vi "Z900_navX_Internal_UpdateDevice.vi"(8 "error in (no error)":errorcluster, 10 "Interface TypeDefs":T1 {"I2CDevRef"."Device Address" format="%.0x"}, 11 "navX Device":T8={"Interface"={"Protocol"=enum."SERIAL", "Update Rate (4Hz-60Hz)"=4, "navX Open TypeDef"=variant}, "Notify Packet"=refnum, "Loop VI Refnum"=refnum} {"Interface"."Update Rate (4Hz-60Hz)" min=4 max=60 step=1}) -> (0 "error out":errorcluster, 2 "Interface TypeDefs":T1 {"I2CDevRef"."Device Address" format="%.0x"}, 3 "navX Device":T8={"Interface"={"Protocol"=enum."SERIAL", "Update Rate (4Hz-60Hz)"=4, "navX Open TypeDef"=variant}, "Notify Packet"=refnum, "Loop VI Refnum"=refnum} {"Interface"."Update Rate (4Hz-60Hz)" min=4 max=60 step=1})   [LabVIEW 2014, in "navX Library v2.lvlib"]
uses:
  navX Library v2.lvlib
  TypeDefs/Z900_navX_DeviceTypeDef.ctl
  TypeDefs/Z900_navX_ProtocolTypeDef.ctl
  TypeDefs/Z900_navX_NotifyPacketTypeDef.ctl
  TypeDefs/Z900_navX_ActionTypeDef.ctl
  TypeDefs/Z900_navX_InterfaceTypeDef.ctl
  <vilib>/Rock Robotics/WPI/SerialPort/WPI_SerialPortRef.ctl
  <vilib>/Rock Robotics/WPI/I2C/WPI_I2CDevRef.ctl
  <vilib>/Rock Robotics/SystemInterfaces/Typedef/FPGA_TypedefDigitalModule.ctl
  <vilib>/Rock Robotics/SystemInterfaces/i2clib/i2c_bus.ctl
  <vilib>/Rock Robotics/WPI/SPI/WPI_SPIDevRef.ctl
  <vilib>/Rock Robotics/SystemInterfaces/spilib/spi_bus.ctl
  TypeDefs/navX Open TypeDefs/Z900_navX_OpenTypeDef_Serial.ctl
  NI WPI/WPI_SerialPort_USB.ctl
  TypeDefs/Z900_navX_SerialStreamTypeDef.ctl
  TypeDefs/navX Open TypeDefs/Z900_navX_OpenTypeDef_I2C.ctl
  TypeDefs/Z900_navX_DeviceRegisters.ctl
  TypeDefs/navX Open TypeDefs/Z900_navX_OpenTypeDef_SPI.ctl
  NI WPI/NI WPI Serial USB.lvlib
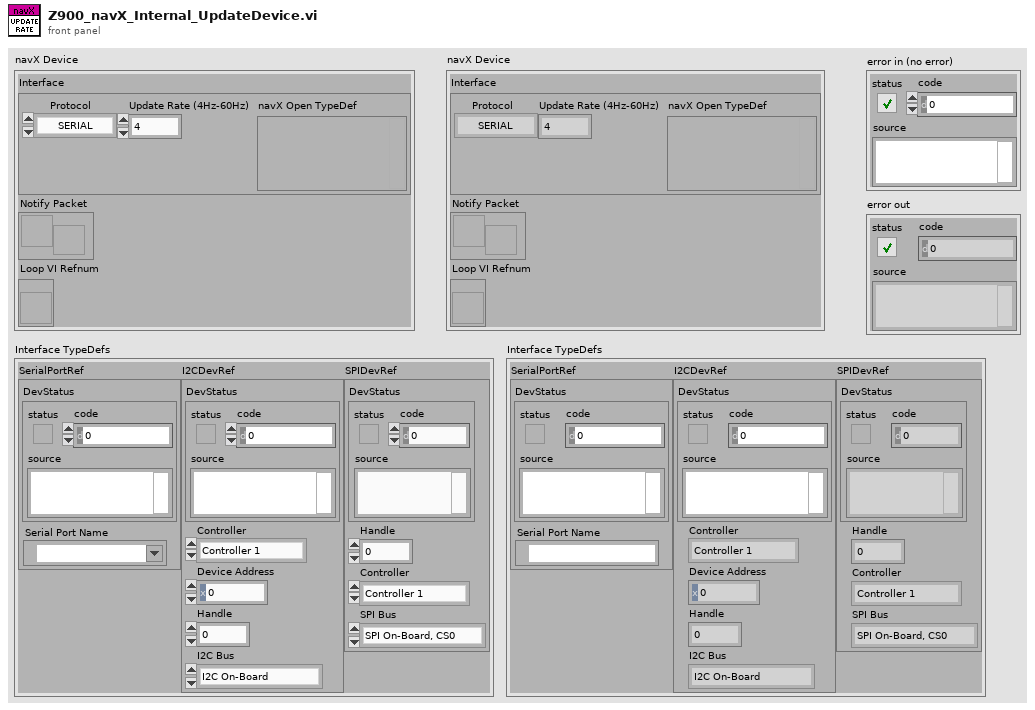
[diagram p1: front panel]
types:
  T1 = typedef "navX Library v2.lvlib/Z900_navX_InterfaceTypeDef.ctl" = cluster{"SerialPortRef":T2, "I2CDevRef":T3, "SPIDevRef":T6}
  T2 = typedef "WPI_SerialPortRef.ctl" = cluster{"DevStatus":errorcluster, "Serial Port Name":refnum<visa-resource-name>}
  T3 = typedef "WPI_I2CDevRef.ctl" = cluster{"DevStatus":errorcluster, "Controller":T4, "Device Address":u8, "Handle":i32, "I2C Bus":T5}
  T4 = typedef "FPGA_TypedefDigitalModule.ctl" = enum16{"Controller 1"}
  T5 = typedef "i2c_bus.ctl" = enum16{"I2C On-Board", "I2C MXP", "Invalid"}
  T6 = typedef "WPI_SPIDevRef.ctl" = cluster{"DevStatus":errorcluster, "Handle":i32, "Controller":T4, "SPI Bus":T7}
  T7 = typedef "spi_bus.ctl" = enum16{"SPI On-Board, CS0", "SPI On-Board, CS1", "SPI On-Board, CS2", "SPI On-Board, CS3", "SPI MXP", "Invalid"}
  T8 = typedef "navX Library v2.lvlib/Z900_navX_DeviceTypeDef.ctl" = cluster{"Interface":cluster{"Protocol":T9, "Update Rate (4Hz-60Hz)":u8, "navX Open TypeDef":variant}, "Notify Packet":refnum<notifier>, "Loop VI Refnum":refnum<vi>}
  T9 = typedef "navX Library v2.lvlib/Z900_navX_ProtocolTypeDef.ctl" = enum16{"SERIAL", "I2C", "SPI"}
  T10 = typedef "navX Library v2.lvlib/Z900_navX_OpenTypeDef_Serial.ctl" = cluster{"Serial Port":T11, "Stream Type":T12}
  T11 = typedef "NI WPI Serial USB.lvlib/WPI_SerialPort_USB.ctl" = enum16{"Onboard RS-232", "MXP TTL", "USB"}
  T12 = typedef "navX Library v2.lvlib/Z900_navX_SerialStreamTypeDef.ctl" = enum16{"YRPH", "Quadernion", "Gyro/Raw", "AHRS", "AHRSAndPositioning"}
  T13 = typedef "navX Library v2.lvlib/Z900_navX_OpenTypeDef_I2C.ctl" = cluster{"I2C Bus":T5}
  T14 = typedef "navX Library v2.lvlib/Z900_navX_OpenTypeDef_SPI.ctl" = cluster{"SPI Bus":T7}
  T15 = typedef "navX Library v2.lvlib/Z900_navX_DeviceRegisters.ctl" = u8
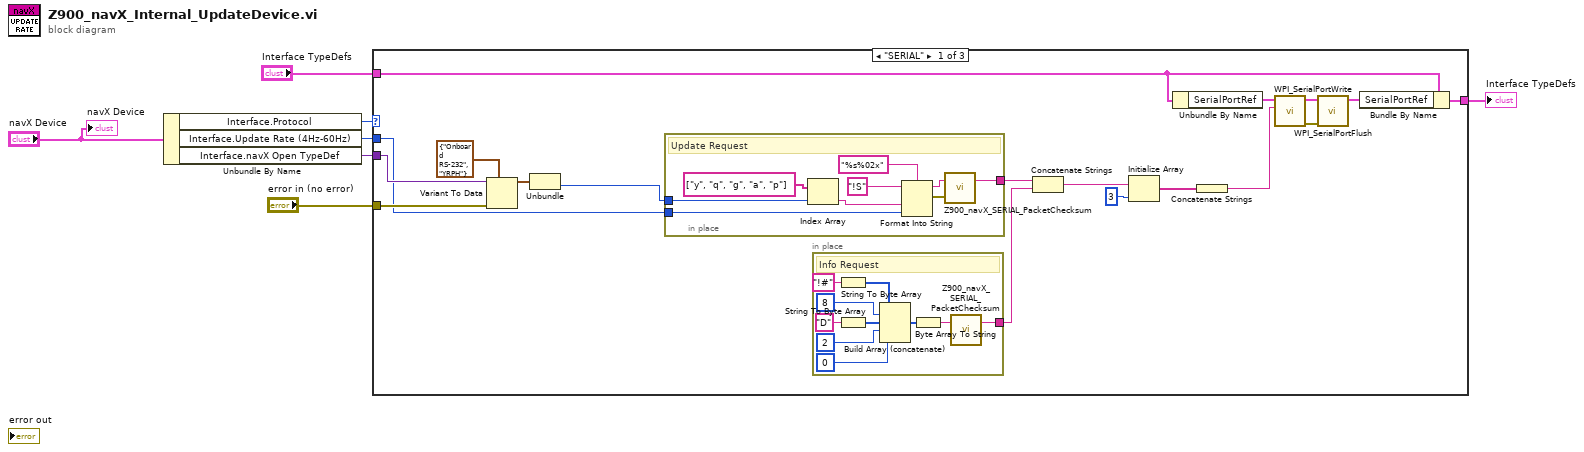
[diagram p0: block diagram]
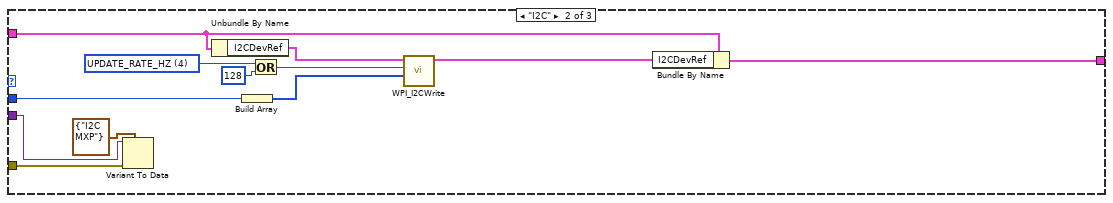
[diagram p2: hidden frame]
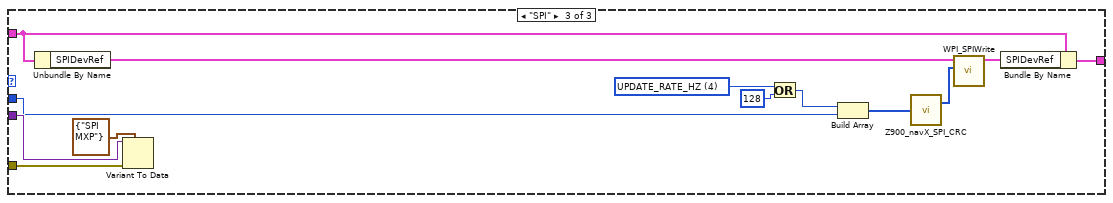
[diagram p3: hidden frame]
diagram:
  n1 = Unbundle By Name("navX Device") -> ("Interface.Protocol"=w6:T9, "Interface.Update Rate (4Hz-60Hz)"=w2:u8, "Interface.navX Open TypeDef"=w5:variant)
  n2 = case shown="\"SERIAL\"" w6 {
    tunnel: w5 -> [w25 w56 w69]
    tunnel: "error in (no error)" -> [w23 w54 w67]
    tunnel: "Interface TypeDefs" -> [w20 w47 w59]
    tunnel: w2 -> [w18 w50 w61]
    tunnel: [w19 w45 w57] -> w1
    frame "SERIAL" {
      n3 = Variant To Data(error in=w23, type=T10 {"Serial Port"=enum."Onboard RS-232", "Stream Type"=enum."YRPH"} ("navX Serial Open"), Variant=w25) -> (data=w22:T10)  [unwired: 1 out]
      n4 = Unbundle(w22) -> ("Stream Type"=w21:T12)  [unwired: 1 out]
      n5 = in-place {
        in-place-border: w21 -> [w33]
        in-place-border: [w32] -> w11
        in-place-border: w18 -> [w26]
        # "Update Request"
        n6 = Index Array(array=string[] ["y", "q", "g", "a", "p"], index=w33) -> (element=w27:string)
        n7 = Format Into String(format string="%s%02x", initial string="!S", w27, w26) -> (resulting string=w30:string, error out=w31:errorcluster)  [unwired: 1 in]
        n8 = call "Z900_navX_SERIAL_PacketChecksum.vi"("error in (no error)"=w31, "Packet"=w30) -> ("Terminated Packet"=w32:string)  [unwired: 1 out]
      }
      n9 = in-place {
        in-place-border: [w35] -> w10
        # "Info Request"
        n10 = String To Byte Array(string="!#" ("initial string")) -> (unsigned byte array=w42:u8[])
        n11 = String To Byte Array(string="D" ("initial string")) -> (unsigned byte array=w40:u8[])
        n12 = Build Array (concatenate)(w42, 8, w40, 2, 0) -> (w37:i32[])
        n13 = Byte Array To String(unsigned byte array=w37) -> (string=w36:string)
        n14 = call "Z900_navX_SERIAL_PacketChecksum.vi"("Packet"=w36) -> ("Terminated Packet"=w35:string)  [unwired: 1 in, 1 out]
      }
      n15 = Concatenate Strings(w11, w10) -> (w9:string)
      n16 = Initialize Array(w9, 3 ("dimension size")) -> (w8:string[])
      n17 = Unbundle By Name(w20) -> ("SerialPortRef"=w16:T2)
      n18 = Concatenate Strings(w8) -> (w12:string)
      n19 = call <vilib>:"WPI_SerialPortWrite.vi"("Buffer"=w12, "SerialPortRef"=w16) -> ("error out"=w14:errorcluster, "SerialPortRef"=w13:T2)  [unwired: 7 in, 1 out]
      n20 = call <vilib>:"WPI_SerialPortFlush.vi"("error in (no error)"=w14, "SerialPortRef"=w13) -> ("SerialPortRef"=w15:T2)  [unwired: 8 in, 1 out]
      n21 = Bundle By Name(cluster=w20, "SerialPortRef"=w15) -> (w19:T1)
    }
    frame "I2C" {
      w51 = T15 4 items=["WHOAMI"=0, "HW_REV"=1, "FW_VER_MAJOR"=2, "FW_VER_MINOR"=3, "UPDATE_RATE_HZ"=4, "ACCEL_FSR_G"=5, "GYRO_FSR_DPS"=6, "OP_STATUS"=8, "CAL_STATUS"=9, "SELFTEST_STATUS"=10, "CAPABILITY_FLAGS_L"=11, "CAPABILITY_FLAGS_H"=12, "SENSOR_STATUS"=16, "TIMESTAMP"=18, "YAW"=22, "ROLL"=24, "PITCH"=26, "HEADING"=28, "FUSED_HEADING"=30, "ALTITUDE_I"=32, "ALTITUDE_D"=34, "LINERA_ACC_X"=36, "LINERA_ACC_Y"=38, "LINERA_ACC_Z"=40, "QUAT_W"=42, "QUAT_X"=44, "QUAT_Y"=46, "QUAT_Z"=48, "MPU_TEMP_C"=50, "GYRO_X"=52, "GYRO_Y"=54, "GYRO_Z"=56, "ACC_X"=58, "ACC_Y"=60, "ACC_Z"=62, "MAG_X"=64, "MAG_Y"=66, "MAG_Z"=68, "PRESSURE_I"=70, "PRESSURE_D"=72, "PRESSURE_TEMP"=74, "YAW_OFFSET"=76, "QUAT_OFFSET_W"=78, "QUAT_OFFSET_X"=80, "QUAT_OFFSET_Y"=82, "QUAT_OFFSET_Z"=84, "INTEGRATION_CONTROL"=86, "VELOCITY_X"=88, "VELOCITY_Y"=92, "VELOCITY_Z"=96, "DISPLACMENT_X"=100, "DISPLACMENT_Y"=104, "DISPLACEMENT_Z"=108] ("Device Register")
      n22 = Variant To Data(error in=w54, type=T13 {"I2C Bus"=enum."I2C MXP"} ("navX I2C Open"), Variant=w56) -> ()  [unwired: 2 out]
      n23 = Unbundle By Name(w47) -> ("I2CDevRef"=w48:T3)
      n24 = Build Array(w50) -> (w49:u8[])
      n25 = Or(x=w51, y=u8 128) -> (x .or. y?=w53:T15)
      n26 = call <vilib>:"WPI_I2CWrite.vi"("I2CDataToSend"=w49, "I2CRegister"=w53, "I2CDevRef"=w48) -> ("I2CDevRef"=w46:T3)  [unwired: 7 in, 1 out]
      n27 = Bundle By Name(cluster=w47, "I2CDevRef"=w46) -> (w45:T1)
    }
    frame "SPI" {
      w63 = T15 4 items=["WHOAMI"=0, "HW_REV"=1, "FW_VER_MAJOR"=2, "FW_VER_MINOR"=3, "UPDATE_RATE_HZ"=4, "ACCEL_FSR_G"=5, "GYRO_FSR_DPS"=6, "OP_STATUS"=8, "CAL_STATUS"=9, "SELFTEST_STATUS"=10, "CAPABILITY_FLAGS_L"=11, "CAPABILITY_FLAGS_H"=12, "SENSOR_STATUS"=16, "TIMESTAMP"=18, "YAW"=22, "ROLL"=24, "PITCH"=26, "HEADING"=28, "FUSED_HEADING"=30, "ALTITUDE_I"=32, "ALTITUDE_D"=34, "LINERA_ACC_X"=36, "LINERA_ACC_Y"=38, "LINERA_ACC_Z"=40, "QUAT_W"=42, "QUAT_X"=44, "QUAT_Y"=46, "QUAT_Z"=48, "MPU_TEMP_C"=50, "GYRO_X"=52, "GYRO_Y"=54, "GYRO_Z"=56, "ACC_X"=58, "ACC_Y"=60, "ACC_Z"=62, "MAG_X"=64, "MAG_Y"=66, "MAG_Z"=68, "PRESSURE_I"=70, "PRESSURE_D"=72, "PRESSURE_TEMP"=74, "YAW_OFFSET"=76, "QUAT_OFFSET_W"=78, "QUAT_OFFSET_X"=80, "QUAT_OFFSET_Y"=82, "QUAT_OFFSET_Z"=84, "INTEGRATION_CONTROL"=86, "VELOCITY_X"=88, "VELOCITY_Y"=92, "VELOCITY_Z"=96, "DISPLACMENT_X"=100, "DISPLACMENT_Y"=104, "DISPLACEMENT_Z"=108] ("Device Register")
      n28 = Unbundle By Name(w59) -> ("SPIDevRef"=w60:T6)
      n29 = Variant To Data(error in=w67, type=T14 {"SPI Bus"=enum."SPI MXP"} ("navX SPI Open"), Variant=w69) -> ()  [unwired: 2 out]
      n30 = Or(x=w63, y=u8 128) -> (x .or. y?=w64:T15)
      n31 = Build Array(w64, w61) -> (w65:T15[])
      n32 = call "Z900_navX_SPI_CRC.vi"("Message"=w65) -> ("Message with CRC"=w66:u8[])  [unwired: 1 out]
      n33 = call <vilib>:"WPI_SPIWrite.vi"("Data To Send"=w66, "SPIDevRef"=w60) -> ("SPIDevRef"=w58:T6)  [unwired: 7 in, 2 out]
      n34 = Bundle By Name(cluster=w59, "SPIDevRef"=w58) -> (w57:T1)
    }
  }
  "Interface TypeDefs" <- w1
  "navX Device" <- "navX Device"
